vi "Create a control from variant.vi"(4 "Terminal Position":T1, 5 "Terminal Source/Sink":refnum<vi>, 6 "FP position":T1, 7 "Indicator?":bool, 8 "error in (no error)":errorcluster, 10 "Constant Data":variant, 11 "Diagram":refnum<vi>) -> (0 "error out":errorcluster, 2 "Terminal":refnum<vi>, 3 "Control Reference":refnum<vi>)   [LabVIEW 2012, in "Scripting Tools.lvlib"]
doc: "Create a constant on the block diagram with name and type of <b>Constant Data</b>."
uses:
  Scripting Tools.lvlib
  <vilib>/Utility/miscctls.llb/LVPointTypeDef.ctl
  <vilib>/Utility/VariantDataType/VariantType.lvlib
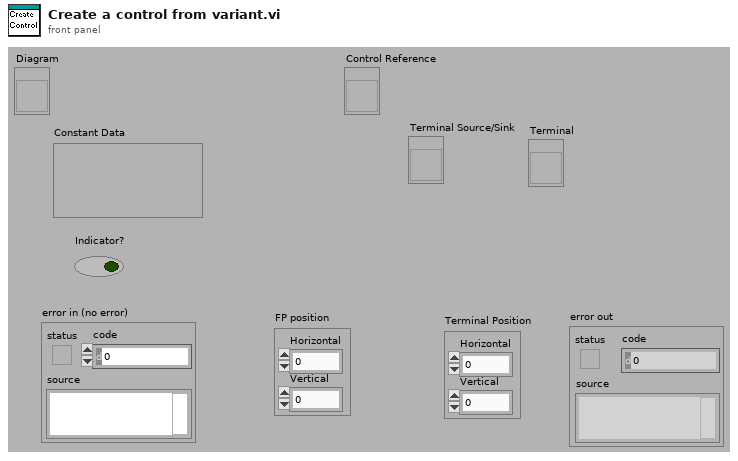
[diagram p1: front panel]
types:
  T1 = typedef "LVPointTypeDef.ctl" = cluster{"Horizontal":i16, "Vertical":i16}
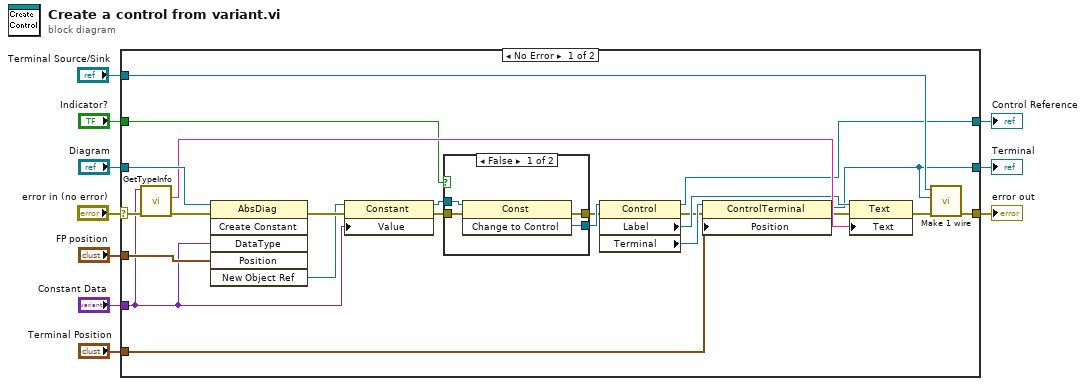
[diagram p0: block diagram]
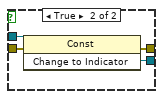
[diagram p2: hidden frame]
diagram:
  n1 = case shown="No Error" "error in (no error)" {
    selector: "error in (no error)" -> [w28 w42]
    tunnel: [w33 w42] -> w9
    tunnel: "Constant Data" -> [w26 _]
    tunnel: "FP position" -> [w31 _]
    tunnel: "Terminal Source/Sink" -> [w18 _]
    tunnel: "Diagram" -> [w32 _]
    tunnel: "Indicator?" -> [w24 _]
    tunnel: [w17 _] -> w3
    tunnel: [w12 _] -> w2
    tunnel: "Terminal Position" -> [w11 _]
    frame No Error {
      n2 = call <vilib>:"GetTypeInfo.vi"("error in (no error)"=w28, "Variant"=w26) -> ("error out"=w27:errorcluster, "Name"=w25:string)  [unwired: 8 out]
      n3 = invoke class="AbsDiag" method="Create Constant"(reference=w32, error in=w27, "DataType"=w26, "Position"=w31) -> (error out=w30:errorcluster, "New Object Ref"=w29:refnum<vi>)  [unwired: 2 in, 4 out]
      n4 = property class="Constant"(reference=w29, error in=w30, "Value"=w26) -> (reference out=w22:refnum<vi>, error out=w23:errorcluster)
      n5 = case shown="False" w24 {
        tunnel: w23 -> [w36 w41]
        tunnel: w22 -> [w37 w40]
        tunnel: [w34 w39] -> w21
        tunnel: [w35 w38] -> w20
        frame False {
          n6 = invoke class="Const" method="Change to Control"(reference=w37, error in=w36) -> (error out=w35:errorcluster, "Change to Control"=w34:refnum<vi>)  [unwired: 1 in, 1 out]
        }
        frame True {
          n7 = invoke class="Const" method="Change to Indicator"(reference=w40, error in=w41) -> (error out=w38:errorcluster, "Change to Indicator"=w39:refnum<vi>)  [unwired: 1 in, 1 out]
        }
      }
      n8 = property class="Control"(reference=w21, error in=w20) -> (reference out=w17:refnum<vi>, error out=w14:errorcluster, "Label"=w19:refnum<vi>, "Terminal"=w15:refnum<vi>)
      n9 = property class="ControlTerminal"(reference=w15, error in=w14, "Position"=w11) -> (reference out=w12:refnum<vi>, error out=w13:errorcluster)
      n10 = property class="Text"(reference=w19, error in=w13, "Text"=w25) -> (error out=w16:errorcluster)  [unwired: 1 out]
      n11 = call "Make 1 wire.vi"("error in"=w16, "Wire Terminal 2"=w12, "Wire Terminal 1"=w18) -> ("error out"=w33:errorcluster)  [unwired: 8 out]
    }
    frame Error {
    }
  }
  "error out" <- w9
  "Control Reference" <- w3
  "Terminal" <- w2
